vi "Processing Step.vi"(8 "error in (no error)":errorcluster, 11 "WebSocket Handler in":refnum<class "WebSocket Handler.lvclass">) -> (0 "error out":errorcluster, 2 "Array":T1[](array[typedef]), 3 "WebSocket Handler out":refnum<class "WebSocket Handler.lvclass">)   [LabVIEW 2020, in "HTTP Server.lvlib" / "WebSocket Handler.lvclass"]
uses:
  WebSocket Handler.lvclass
  Processing Step.ctl
  HTTP Server.lvlib
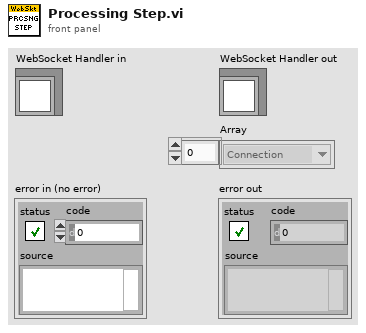
[diagram p1: front panel]
types:
  T1 = typedef "HTTP Server.lvlib/Processing Step.ctl" = enum16{"Connection", "Request", "Routing", "Controller Init", "Controller", "Response", "Complete", "Exception"}
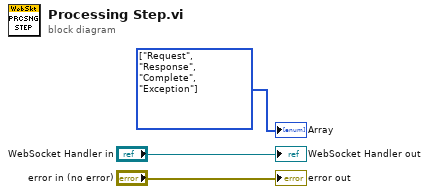
[diagram p0: block diagram]
diagram:
  w1 = T1[] [enum."Request", enum."Response", enum."Complete", enum."Exception"] items=["Connection", "Request", "Routing", "Controller Init", "Controller", "Response", "Complete", "Exception"] ("Array")
  "error out" <- "error in (no error)"
  "WebSocket Handler out" <- "WebSocket Handler in"
  "Array" <- w1
